vi "S4GUI.vi"() -> ()   [LabVIEW 2018] (continued)
                n1589 = call-dynamic "Write Interface.vi"("error in (no error)"=w3557, "Interface.lvclass"=w3544, "Channel in"=w3552) -> ("error out"=w3525:errorcluster, "Channel out"=w3524:refnum<class "Channel.lvclass">)  [unwired: 7 in]
                n1590 = call-dynamic "Write ciclos.vi"("error in (no error)"=w3525, "ciclos"=w3523, "Channel in"=w3524) -> ("error out"=w3521:errorcluster, "Channel out"=w3522:refnum<class "Channel.lvclass">)  [unwired: 7 in]
                n1591 = call-dynamic "Write sequencias.vi"("error in (no error)"=w3521, "sequencias"=w3518, "Channel in"=w3522) -> ("error out"=w3520:errorcluster, "Channel out"=w3519:refnum<class "Channel.lvclass">)  [unwired: 7 in]
                n1592 = call-dynamic "Write Channel.vi"("error in (no error)"=w3520, "Channel.lvclass"=w3519, "Acquisition in"=w3542) -> ("error out"=w3540:errorcluster, "Acquisition out"=w3541:refnum<class "Acquisition.lvclass">)  [unwired: 7 in]
                n1593 = call-dynamic "Write AcquisitionD.vi"("error in (no error)"=w3540, "Acquisition.lvclass"=w3541, "S4ACS_GUI in"=w3543) -> ("error out"=w3566:errorcluster, "S4ACS_GUI out"=w3567:refnum<class "S4GUI.lvclass">)  [unwired: 7 in]
              }
            }
            n1594 = call-dynamic "Write sequencias.vi"("error in (no error)"=w3342, "sequencias"=w3338, "S4GUI in"=w3340) -> ("error out"=w3341:errorcluster, "S4GUI out"=w3339:refnum<class "S4GUI.lvclass">)  [unwired: 7 in]
            n1595 = call-dynamic "Write ciclos.vi"("error in (no error)"=w3341, "ciclos"=w3343, "S4ACS_GUI in"=w3339) -> ("error out"=w3345:errorcluster, "S4ACS_GUI out"=w3347:refnum<class "S4GUI.lvclass">)  [unwired: 7 in]
            n1596 = property on="#Cycles Done" class="Slide (strict)"("Scale.Maximum"=w3343, "Scale.Minimum"=0.0 ("Scale.Range:Minor Increment")) -> ()  [unwired: 2 in, 2 out]
            n1597 = call-dynamic "Write TotalCiclos.vi"("error in (no error)"=w3345, "TotalCiclos"=w3343, "S4GUI in"=w3347) -> ("error out"=w3344:errorcluster, "S4GUI out"=w3346:refnum<class "S4GUI.lvclass">)  [unwired: 7 in]
          }
        }
        n1598 = property on="Pause SM" class="Bool"(error in=w3207, "DisabledEnum"=T7."Enabled" ("Disabled")) -> (error out=w3206:errorcluster)  [unwired: 1 in, 1 out]
      }
      event "# Cycles": Value Change {
        n1599 = event-data() -> ("NewVal"=w3572:u32)  [unwired: 1 in]
        n1600 = call-dynamic "Write ciclos.vi"("error in (no error)"=w3573, "ciclos"=w3572, "S4ACS_GUI in"=w3574) -> ("error out"=w3571:errorcluster, "S4ACS_GUI out"=w3570:refnum<class "S4GUI.lvclass">)  [unwired: 7 in]
        n1601 = property on="#Cycles Done" class="Slide (strict)"("Scale.Maximum"=w3572, "Scale.Minimum"=0.0 ("Scale.Range:Minor Increment")) -> ()  [unwired: 2 in, 2 out]
      }
      event "AllConfig": Value Change {
        n1602 = event-data() -> ()  [unwired: 1 in, 6 out]
        n1603 = call "Read Instrument.lvclass.vi"("error in (no error)"=w3580, "S4ACS_GUI in"=w3581) -> ("error out"=w3660:errorcluster, "Instrument.lvclass"=w3627:refnum<class "Instrument.lvclass">, "S4ACS_GUI out"=w3658:refnum<class "S4GUI.lvclass">)  [unwired: 7 in]
        n1604 = call "Read ASEL.vi"("error in (no error)"=w3660, "Instrument in"=w3627) -> ("error out"=w3652:errorcluster, "Opt_Selector.lvclass"=w3651:refnum<class "Opt_Selector.lvclass">, "Instrument out"=w3659:refnum<class "Instrument.lvclass">)  [unwired: 7 in]
        n1605 = call-dynamic "Read State Machine.vi"("error in (no error)"=w3652, "Device in"=w3651) -> ("error out"=w3655:errorcluster, "State Machine.lvclass"=w3657:refnum<class "State Machine.lvclass">, "Device out"=w3649:refnum<class "Opt_Selector.lvclass">)  [unwired: 7 in]
        n1606 = call "Next State.vi"("error in (no error)"=w3655, "New_State"=1, "State Machine in"=w3657) -> ("error out"=w3654:errorcluster, "State Machine out"=w3653:refnum<class "State Machine.lvclass">)  [unwired: 7 in]
        n1607 = call-dynamic "Write State Machine.vi"("error in (no error)"=w3654, "State Machine.lvclass"=w3653, "Device in"=w3649) -> ("error out"=w3648:errorcluster, "Device out"=w3650:refnum<class "Opt_Selector.lvclass">)  [unwired: 7 in]
        n1608 = call "Write ASEL.vi"("error in (no error)"=w3648, "Opt_Selector.lvclass"=w3650, "Instrument in"=w3659) -> ("error out"=w3610:errorcluster, "Instrument out"=w3626:refnum<class "Instrument.lvclass">)  [unwired: 7 in]
        n1609 = call "Read CALW.vi"("error in (no error)"=w3610, "Instrument in"=w3626) -> ("error out"=w3643:errorcluster, "Opt_Selector.lvclass"=w3644:refnum<class "Opt_Selector.lvclass">, "Instrument out"=w3625:refnum<class "Instrument.lvclass">)  [unwired: 7 in]
        n1610 = call-dynamic "Read State Machine.vi"("error in (no error)"=w3643, "Device in"=w3644) -> ("error out"=w3640:errorcluster, "State Machine.lvclass"=w3638:refnum<class "State Machine.lvclass">, "Device out"=w3646:refnum<class "Opt_Selector.lvclass">)  [unwired: 7 in]
        n1611 = call "Next State.vi"("error in (no error)"=w3640, "New_State"=1, "State Machine in"=w3638) -> ("error out"=w3641:errorcluster, "State Machine out"=w3642:refnum<class "State Machine.lvclass">)  [unwired: 7 in]
        n1612 = call-dynamic "Write State Machine.vi"("error in (no error)"=w3641, "State Machine.lvclass"=w3642, "Device in"=w3646) -> ("error out"=w3647:errorcluster, "Device out"=w3645:refnum<class "Opt_Selector.lvclass">)  [unwired: 7 in]
        n1613 = call "Write CALW.vi"("error in (no error)"=w3647, "Opt_Selector.lvclass"=w3645, "Instrument in"=w3625) -> ("error out"=w3609:errorcluster, "Instrument out"=w3624:refnum<class "Instrument.lvclass">)  [unwired: 7 in]
        n1614 = call "Read WPSEL.vi"("error in (no error)"=w3609, "Instrument in"=w3624) -> ("error out"=w3632:errorcluster, "Opt_Selector.lvclass"=w3631:refnum<class "Opt_Selector.lvclass">, "Instrument out"=w3623:refnum<class "Instrument.lvclass">)  [unwired: 7 in]
        n1615 = call-dynamic "Read State Machine.vi"("error in (no error)"=w3632, "Device in"=w3631) -> ("error out"=w3635:errorcluster, "State Machine.lvclass"=w3637:refnum<class "State Machine.lvclass">, "Device out"=w3629:refnum<class "Opt_Selector.lvclass">)  [unwired: 7 in]
        n1616 = call "Next State.vi"("error in (no error)"=w3635, "New_State"=1, "State Machine in"=w3637) -> ("error out"=w3634:errorcluster, "State Machine out"=w3633:refnum<class "State Machine.lvclass">)  [unwired: 7 in]
        n1617 = call-dynamic "Write State Machine.vi"("error in (no error)"=w3634, "State Machine.lvclass"=w3633, "Device in"=w3629) -> ("error out"=w3628:errorcluster, "Device out"=w3630:refnum<class "Opt_Selector.lvclass">)  [unwired: 7 in]
        n1618 = call "Write WPSEL.vi"("error in (no error)"=w3628, "Opt_Selector.lvclass"=w3630, "Instrument in"=w3623) -> ("error out"=w3608:errorcluster, "Instrument out"=w3612:refnum<class "Instrument.lvclass">)  [unwired: 7 in]
        n1619 = call "Read WPROT.vi"("error in (no error)"=w3608, "Instrument in"=w3612) -> ("error out"=w3618:errorcluster, "Opt_Selector.lvclass"=w3619:refnum<class "Opt_Selector.lvclass">, "Instrument out"=w3611:refnum<class "Instrument.lvclass">)  [unwired: 7 in]
        n1620 = call-dynamic "Read State Machine.vi"("error in (no error)"=w3618, "Device in"=w3619) -> ("error out"=w3615:errorcluster, "State Machine.lvclass"=w3613:refnum<class "State Machine.lvclass">, "Device out"=w3621:refnum<class "Opt_Selector.lvclass">)  [unwired: 7 in]
        n1621 = call "Next State.vi"("error in (no error)"=w3615, "New_State"=1, "State Machine in"=w3613) -> ("error out"=w3616:errorcluster, "State Machine out"=w3617:refnum<class "State Machine.lvclass">)  [unwired: 7 in]
        n1622 = call-dynamic "Write State Machine.vi"("error in (no error)"=w3616, "State Machine.lvclass"=w3617, "Device in"=w3621) -> ("error out"=w3622:errorcluster, "Device out"=w3620:refnum<class "Opt_Selector.lvclass">)  [unwired: 7 in]
        n1623 = call "Write WPROT.vi"("error in (no error)"=w3622, "Opt_Selector.lvclass"=w3620, "Instrument in"=w3611) -> ("error out"=w3584:errorcluster, "Instrument out"=w3585:refnum<class "Instrument.lvclass">)  [unwired: 7 in]
        n1624 = call "Read GMIR.vi"("error in (no error)"=w3584, "Instrument in"=w3585) -> ("error out"=w3603:errorcluster, "Opt_Continuous.lvclass"=w3604:refnum<class "Opt_Continuous.lvclass">, "Instrument out"=w3597:refnum<class "Instrument.lvclass">)  [unwired: 7 in]
        n1625 = call-dynamic "Read State Machine.vi"("error in (no error)"=w3603, "Device in"=w3604) -> ("error out"=w3600:errorcluster, "State Machine.lvclass"=w3598:refnum<class "State Machine.lvclass">, "Device out"=w3606:refnum<class "Opt_Continuous.lvclass">)  [unwired: 7 in]
        n1626 = call "Next State.vi"("error in (no error)"=w3600, "New_State"=1, "State Machine in"=w3598) -> ("error out"=w3601:errorcluster, "State Machine out"=w3602:refnum<class "State Machine.lvclass">)  [unwired: 7 in]
        n1627 = call-dynamic "Write State Machine.vi"("error in (no error)"=w3601, "State Machine.lvclass"=w3602, "Device in"=w3606) -> ("error out"=w3607:errorcluster, "Device out"=w3605:refnum<class "Opt_Continuous.lvclass">)  [unwired: 7 in]
        n1628 = call "Write GMIR.vi"("error in (no error)"=w3607, "Opt_Continuous.lvclass"=w3605, "Instrument in"=w3597) -> ("error out"=w3582:errorcluster, "Instrument out"=w3583:refnum<class "Instrument.lvclass">)  [unwired: 7 in]
        n1629 = call "Read GFOC.vi"("error in (no error)"=w3582, "Instrument in"=w3583) -> ("error out"=w3592:errorcluster, "Opt_Continuous.lvclass"=w3593:refnum<class "Opt_Continuous.lvclass">, "Instrument out"=w3586:refnum<class "Instrument.lvclass">)  [unwired: 7 in]
        n1630 = call-dynamic "Read State Machine.vi"("error in (no error)"=w3592, "Device in"=w3593) -> ("error out"=w3589:errorcluster, "State Machine.lvclass"=w3587:refnum<class "State Machine.lvclass">, "Device out"=w3595:refnum<class "Opt_Continuous.lvclass">)  [unwired: 7 in]
        n1631 = call "Next State.vi"("error in (no error)"=w3589, "New_State"=1, "State Machine in"=w3587) -> ("error out"=w3590:errorcluster, "State Machine out"=w3591:refnum<class "State Machine.lvclass">)  [unwired: 7 in]
        n1632 = call-dynamic "Write State Machine.vi"("error in (no error)"=w3590, "State Machine.lvclass"=w3591, "Device in"=w3595) -> ("error out"=w3596:errorcluster, "Device out"=w3594:refnum<class "Opt_Continuous.lvclass">)  [unwired: 7 in]
        n1633 = call "Write GFOC.vi"("error in (no error)"=w3596, "Opt_Continuous.lvclass"=w3594, "Instrument in"=w3586) -> ("error out"=w3578:errorcluster, "Instrument out"=w3579:refnum<class "Instrument.lvclass">)  [unwired: 7 in]
        n1634 = call "Write Instrument.lvclass.vi"("error in (no error)"=w3578, "Instrument.lvclass"=w3579, "S4ACS_GUI in"=w3658) -> ("error out"=w3577:errorcluster, "S4ACS_GUI out"=w3576:refnum<class "S4GUI.lvclass">)  [unwired: 7 in]
      }
      event "Tab Acq Type": Value Change {
        # "Tab for choosing EXPOSURE MODE: Object, Dflat, Sflat, Dark, Zero, Focus"
        n1635 = event-data() -> ("NewVal"=w3667:T1)  [unwired: 1 in]
        n1636 = local read "Observer"() -> (w3662:string)
        n1637 = case shown="\"OBJECT\", Default" w3667 {
          tunnel: ["OBJECT" "FLAT" "FLAT" "DARK" "ZERO" "FOCUS"] -> w3666
          tunnel: [w3703 w3707 w3711 w3715 w3719 w3723] -> w3665
          tunnel: [w3702 w3706 w3710 w3714 w3718 w3722] -> w3664
          tunnel: [w3701 w3705 w3709 w3713 w3717 w3721] -> w3663
          frame "OBJECT", Default {
            n1638 = local read "Object_obj"() -> (w3703:string)
            n1639 = local read "OBJECT Comments"() -> (w3701:string)
            n1640 = local read "object suffix"() -> (w3702:string)
          }
          frame "DFLAT" {
            n1641 = local read "DFLAT Comments"() -> (w3705:string)
            n1642 = local read "Object_dflat"() -> (w3707:string)
            n1643 = local read "dflat suffix"() -> (w3706:string)
          }
          frame "SFLAT" {
            n1644 = local read "SFLAT Comments"() -> (w3709:string)
            n1645 = local read "Object_sflat"() -> (w3711:string)
            n1646 = local read "sflat suffix"() -> (w3710:string)
          }
          frame "DARK" {
            n1647 = local read "Object_dark"() -> (w3715:string)
            n1648 = local read "dark suffix"() -> (w3714:string)
            n1649 = local read "DARK Comments"() -> (w3713:string)
          }
          frame "ZERO" {
            n1650 = local read "ZERO Comments"() -> (w3717:string)
            n1651 = local read "Object_zero"() -> (w3719:string)
            n1652 = local read "zero suffix"() -> (w3718:string)
          }
          frame "FOCUS" {
            n1653 = local read "FOCUS Comments"() -> (w3721:string)
            n1654 = local read "Object_focus"() -> (w3723:string)
            n1655 = local read "focus suffix"() -> (w3722:string)
          }
        }
        n1656 = call-dynamic "Write ExpMode.vi"("error in (no error)"=w3670, "ExpMode"=w3667, "S4GUI in"=w3671) -> ("error out"=w3668:errorcluster, "S4GUI out"=w3669:refnum<class "S4GUI.lvclass">)  [unwired: 7 in]
        n1657 = call-dynamic "Read AcquisitionC.vi"("error in (no error)"=w3668, "S4ACS_GUI in"=w3669) -> ("error out"=w3674:errorcluster, "Acquisition.lvclass"=w3675:refnum<class "Acquisition.lvclass">)  [unwired: 7 in, 1 out]
        n1658 = call-dynamic "Read AcquisitionA.vi"("error in (no error)"=w3668, "S4ACS_GUI in"=w3669) -> ("error out"=w3678:errorcluster, "Acquisition.lvclass"=w3679:refnum<class "Acquisition.lvclass">, "S4ACS_GUI out"=w3700:refnum<class "S4GUI.lvclass">)  [unwired: 7 in]
        n1659 = call "Read AcquisitionB.vi"("error in (no error)"=w3668, "S4ACS_GUI in"=w3669) -> ("error out"=w3676:errorcluster, "Acquisition.lvclass"=w3677:refnum<class "Acquisition.lvclass">)  [unwired: 7 in, 1 out]
        n1660 = call-dynamic "Read AcquisitionD.vi"("error in (no error)"=w3668, "S4ACS_GUI in"=w3669) -> ("error out"=w3672:errorcluster, "Acquisition.lvclass"=w3673:refnum<class "Acquisition.lvclass">)  [unwired: 7 in, 1 out]
        n1661 = To Lower Case(string=w3664) -> (all lower case string=w3661:string)
        n1662 = case shown="\"OBJECT\", Default" w3667 {
          tunnel: [w3753 w3942 w4136] -> w3699
          tunnel: [w3752 w3941 w4135] -> w3698
          tunnel: [w3751 w3940 w4134] -> w3694
          tunnel: [w3750 w3939 w4133] -> w3693
          tunnel: [w3749 w3938 w4132] -> w3683
          tunnel: [w3748 w3937 w4131] -> w3682
          tunnel: [w3747 w3936 w4130] -> w3681
          tunnel: [w3746 w3935 w4129] -> w3680
          tunnel: w3679 -> [w3745 w3934 w4128]
          tunnel: w3678 -> [w3744 w3933 w4127]
          tunnel: w3677 -> [w3730 w3920 w4114]
          tunnel: w3676 -> [w3729 w3919 w4113]
          tunnel: w3675 -> [w3728 w3918 w4112]
          tunnel: w3674 -> [w3727 w3917 w4111]
          tunnel: w3673 -> [w3726 w3916 w4110]
          tunnel: w3672 -> [w3725 w3915 w4109]
          tunnel: w3661 -> [_ _ w4108]
          tunnel: w3666 -> [_ _ w4107]
          tunnel: w3665 -> [_ _ w4106]
          tunnel: w3663 -> [_ _ w4105]
          tunnel: w3662 -> [_ _ w4104]
          frame "ZERO" {
            w3743 = 1e-05 ("Exptime ch1")
            # "ZERO: EXPTIME=1E-5 (mandatory) and shutter automatically closed."
            n1663 = call "Read connection.vi"("error in (no error)"=w3725, "Server in"=w3726) -> ("error out"=w3732:errorcluster, "connection"=w3731:bool, "Server out"=w3733:refnum<class "Acquisition.lvclass">)  [unwired: 7 in]
            n1664 = call "Read connection.vi"("error in (no error)"=w3727, "Server in"=w3728) -> ("error out"=w3735:errorcluster, "connection"=w3734:bool, "Server out"=w3736:refnum<class "Acquisition.lvclass">)  [unwired: 7 in]
            n1665 = call "Read connection.vi"("error in (no error)"=w3729, "Server in"=w3730) -> ("error out"=w3738:errorcluster, "connection"=w3737:bool, "Server out"=w3739:refnum<class "Acquisition.lvclass">)  [unwired: 7 in]
            n1666 = call "Read connection.vi"("error in (no error)"=w3744, "Server in"=w3745) -> ("error out"=w3741:errorcluster, "connection"=w3740:bool, "Server out"=w3742:refnum<class "Acquisition.lvclass">)  [unwired: 7 in]
            n1667 = case shown="True" w3737 {
              tunnel: w3739 -> [w3838 w3842]
              tunnel: w3738 -> [w3837 w3841]
              tunnel: [w3838 w3840] -> w3751
              tunnel: [w3837 w3839] -> w3750
              frame False {
              }
              frame True {
                # "nome do arquivo .cfg"
                # "seção no arquivo .cfg"
                # "closed"
                n1668 = call-dynamic "Read Channel.vi"("error in (no error)"=w3841, "Acquisition in"=w3842) -> ("error out"=w3846:errorcluster, "Channel.lvclass"=w3845:refnum<class "Channel.lvclass">, "Acquisition out"=w3844:refnum<class "Acquisition.lvclass">)  [unwired: 7 in]
                n1669 = call-dynamic "Read Interface.vi"("error in (no error)"=w3846, "Channel in"=w3845) -> ("error out"=w3854:errorcluster, "Interface.lvclass"=w3855:refnum<class "Interface.lvclass">, "Channel out"=w3843:refnum<class "Channel.lvclass">)  [unwired: 7 in]
                n1670 = call-dynamic "Get CCD_Config.vi"("error in (no error)"=w3854, "Interface in"=w3855) -> ("error out"=w3851:errorcluster, "output cluster"=w3850:T24, "Interface out"=w3856:refnum<class "Interface.lvclass">)  [unwired: 7 in]
                n1671 = Bundle By Name(cluster=w3850, "SHUTTER_MODE"=u8 2) -> (w3852:T24)
                n1672 = call-dynamic "Set CCD_Config.vi"("error in (no error)"=w3851, "input cluster"=w3852, "Interface in"=w3856) -> ("error out"=w3849:errorcluster, "Interface out"=w3857:refnum<class "Interface.lvclass">)  [unwired: 7 in]
                n1673 = Flatten To String(anything=w3852, error in (no error)=w3849) -> (data string=w3847:string, error out=w3848:errorcluster)  [unwired: 2 in, 1 out]
                n1674 = call "Write flatted cluster.vi"("error in (no error)"=w3848, "flatted cluster"=w3847, "Interface in"=w3857) -> ("error out"=w3859:errorcluster, "Interface out"=w3858:refnum<class "Interface.lvclass">)  [unwired: 7 in]
                n1675 = call-dynamic "Write Interface.vi"("error in (no error)"=w3859, "Interface.lvclass"=w3858, "Channel in"=w3843) -> ("error out"=w3865:errorcluster, "Channel out"=w3866:refnum<class "Channel.lvclass">)  [unwired: 7 in]
                n1676 = call "Write section_name.vi"("error in (no error)"=w3865, "section_name"="CCD_ACS2", "Channel in"=w3866) -> ("error out"=w3863:errorcluster, "Channel out"=w3869:refnum<class "Channel.lvclass">)  [unwired: 7 in]
                n1677 = call-dynamic "save config.vi"("error in (no error)"=w3863, "file config"="lastsaved.cfg", "Channel in"=w3869) -> ("error out"=w3864:errorcluster, "Channel out"=w3870:refnum<class "Channel.lvclass">)  [unwired: 7 in]
                n1678 = call-dynamic "Read State Machine.vi"("error in (no error)"=w3864, "Device in"=w3870) -> ("error out"=w3860:errorcluster, "State Machine.lvclass"=w3872:refnum<class "State Machine.lvclass">, "Device out"=w3871:refnum<class "Channel.lvclass">)  [unwired: 7 in]
                n1679 = call-dynamic "Write State.vi"("error in (no error)"=w3860, "State"=60, "State Machine in"=w3872) -> ("error out"=w3861:errorcluster, "State Machine out"=w3873:refnum<class "State Machine.lvclass">)  [unwired: 7 in]
                n1680 = call-dynamic "Write State Machine.vi"("error in (no error)"=w3861, "State Machine.lvclass"=w3873, "Device in"=w3871) -> ("error out"=w3875:errorcluster, "Device out"=w3874:refnum<class "Channel.lvclass">)  [unwired: 7 in]
                n1681 = call-dynamic "Write Channel.vi"("error in (no error)"=w3875, "Channel.lvclass"=w3874, "Acquisition in"=w3844) -> ("error out"=w3839:errorcluster, "Acquisition out"=w3840:refnum<class "Acquisition.lvclass">)  [unwired: 7 in]
              }
            }
            n1682 = case shown="True" w3740 {
              tunnel: [w3876 w3910] -> w3752
              tunnel: [w3877 w3909] -> w3753
              tunnel: w3742 -> [w3877 w3879]
              tunnel: w3741 -> [w3876 w3878]
              frame False {
              }
              frame True {
                # "nome do arquivo .cfg"
                # "seção no arquivo .cfg"
                # "closed"
                n1683 = call-dynamic "Read Channel.vi"("error in (no error)"=w3878, "Acquisition in"=w3879) -> ("error out"=w3911:errorcluster, "Channel.lvclass"=w3912:refnum<class "Channel.lvclass">, "Acquisition out"=w3913:refnum<class "Acquisition.lvclass">)  [unwired: 7 in]
                n1684 = call-dynamic "Read Interface.vi"("error in (no error)"=w3911, "Channel in"=w3912) -> ("error out"=w3901:errorcluster, "Interface.lvclass"=w3900:refnum<class "Interface.lvclass">, "Channel out"=w3914:refnum<class "Channel.lvclass">)  [unwired: 7 in]
                n1685 = call-dynamic "Get CCD_Config.vi"("error in (no error)"=w3901, "Interface in"=w3900) -> ("error out"=w3904:errorcluster, "output cluster"=w3905:T24, "Interface out"=w3899:refnum<class "Interface.lvclass">)  [unwired: 7 in]
                n1686 = Bundle By Name(cluster=w3905, "SHUTTER_MODE"=u8 2) -> (w3903:T24)
                n1687 = call-dynamic "Set CCD_Config.vi"("error in (no error)"=w3904, "input cluster"=w3903, "Interface in"=w3899) -> ("error out"=w3906:errorcluster, "Interface out"=w3898:refnum<class "Interface.lvclass">)  [unwired: 7 in]
                n1688 = Flatten To String(anything=w3903, error in (no error)=w3906) -> (data string=w3908:string, error out=w3907:errorcluster)  [unwired: 2 in, 1 out]
                n1689 = call "Write flatted cluster.vi"("error in (no error)"=w3907, "flatted cluster"=w3908, "Interface in"=w3898) -> ("error out"=w3896:errorcluster, "Interface out"=w3897:refnum<class "Interface.lvclass">)  [unwired: 7 in]
                n1690 = call-dynamic "Write Interface.vi"("error in (no error)"=w3896, "Interface.lvclass"=w3897, "Channel in"=w3914) -> ("error out"=w3891:errorcluster, "Channel out"=w3890:refnum<class "Channel.lvclass">)  [unwired: 7 in]
                n1691 = call "Write section_name.vi"("error in (no error)"=w3891, "section_name"="CCD_ACS1", "Channel in"=w3890) -> ("error out"=w3892:errorcluster, "Channel out"=w3887:refnum<class "Channel.lvclass">)  [unwired: 7 in]
                n1692 = call-dynamic "save config.vi"("error in (no error)"=w3892, "file config"="lastsaved.cfg", "Channel in"=w3887) -> ("error out"=w3880:errorcluster, "Channel out"=w3881:refnum<class "Channel.lvclass">)  [unwired: 7 in]
                n1693 = call-dynamic "Read State Machine.vi"("error in (no error)"=w3880, "Device in"=w3881) -> ("error out"=w3895:errorcluster, "State Machine.lvclass"=w3885:refnum<class "State Machine.lvclass">, "Device out"=w3886:refnum<class "Channel.lvclass">)  [unwired: 7 in]
                n1694 = call-dynamic "Write State.vi"("error in (no error)"=w3895, "State"=60, "State Machine in"=w3885) -> ("error out"=w3894:errorcluster, "State Machine out"=w3884:refnum<class "State Machine.lvclass">)  [unwired: 7 in]
                n1695 = call-dynamic "Write State Machine.vi"("error in (no error)"=w3894, "State Machine.lvclass"=w3884, "Device in"=w3886) -> ("error out"=w3882:errorcluster, "Device out"=w3883:refnum<class "Channel.lvclass">)  [unwired: 7 in]
                n1696 = call-dynamic "Write Channel.vi"("error in (no error)"=w3882, "Channel.lvclass"=w3883, "Acquisition in"=w3913) -> ("error out"=w3910:errorcluster, "Acquisition out"=w3909:refnum<class "Acquisition.lvclass">)  [unwired: 7 in]
              }
            }
            n1697 = case shown="True" w3734 {
              tunnel: w3736 -> [w3799 w3803]
              tunnel: w3735 -> [w3798 w3802]
              tunnel: [w3799 w3801] -> w3749
              tunnel: [w3798 w3800] -> w3748
              frame False {
              }
              frame True {
                # "nome do arquivo .cfg"
                # "seção no arquivo .cfg"
                # "closed"
                n1698 = call-dynamic "Read Channel.vi"("error in (no error)"=w3802, "Acquisition in"=w3803) -> ("error out"=w3807:errorcluster, "Channel.lvclass"=w3806:refnum<class "Channel.lvclass">, "Acquisition out"=w3805:refnum<class "Acquisition.lvclass">)  [unwired: 7 in]
                n1699 = call-dynamic "Read Interface.vi"("error in (no error)"=w3807, "Channel in"=w3806) -> ("error out"=w3815:errorcluster, "Interface.lvclass"=w3816:refnum<class "Interface.lvclass">, "Channel out"=w3804:refnum<class "Channel.lvclass">)  [unwired: 7 in]
                n1700 = call-dynamic "Get CCD_Config.vi"("error in (no error)"=w3815, "Interface in"=w3816) -> ("error out"=w3812:errorcluster, "output cluster"=w3811:T24, "Interface out"=w3817:refnum<class "Interface.lvclass">)  [unwired: 7 in]
                n1701 = Bundle By Name(cluster=w3811, "SHUTTER_MODE"=u8 2) -> (w3813:T24)
                n1702 = call-dynamic "Set CCD_Config.vi"("error in (no error)"=w3812, "input cluster"=w3813, "Interface in"=w3817) -> ("error out"=w3810:errorcluster, "Interface out"=w3818:refnum<class "Interface.lvclass">)  [unwired: 7 in]
                n1703 = Flatten To String(anything=w3813, error in (no error)=w3810) -> (data string=w3808:string, error out=w3809:errorcluster)  [unwired: 2 in, 1 out]
                n1704 = call "Write flatted cluster.vi"("error in (no error)"=w3809, "flatted cluster"=w3808, "Interface in"=w3818) -> ("error out"=w3820:errorcluster, "Interface out"=w3819:refnum<class "Interface.lvclass">)  [unwired: 7 in]
                n1705 = call-dynamic "Write Interface.vi"("error in (no error)"=w3820, "Interface.lvclass"=w3819, "Channel in"=w3804) -> ("error out"=w3826:errorcluster, "Channel out"=w3827:refnum<class "Channel.lvclass">)  [unwired: 7 in]
                n1706 = call "Write section_name.vi"("error in (no error)"=w3826, "section_name"="CCD_ACS3", "Channel in"=w3827) -> ("error out"=w3824:errorcluster, "Channel out"=w3830:refnum<class "Channel.lvclass">)  [unwired: 7 in]
                n1707 = call-dynamic "save config.vi"("error in (no error)"=w3824, "file config"="lastsaved.cfg", "Channel in"=w3830) -> ("error out"=w3825:errorcluster, "Channel out"=w3831:refnum<class "Channel.lvclass">)  [unwired: 7 in]
                n1708 = call-dynamic "Read State Machine.vi"("error in (no error)"=w3825, "Device in"=w3831) -> ("error out"=w3821:errorcluster, "State Machine.lvclass"=w3833:refnum<class "State Machine.lvclass">, "Device out"=w3832:refnum<class "Channel.lvclass">)  [unwired: 7 in]
                n1709 = call-dynamic "Write State.vi"("error in (no error)"=w3821, "State"=60, "State Machine in"=w3833) -> ("error out"=w3822:errorcluster, "State Machine out"=w3834:refnum<class "State Machine.lvclass">)  [unwired: 7 in]
                n1710 = call-dynamic "Write State Machine.vi"("error in (no error)"=w3822, "State Machine.lvclass"=w3834, "Device in"=w3832) -> ("error out"=w3836:errorcluster, "Device out"=w3835:refnum<class "Channel.lvclass">)  [unwired: 7 in]
                n1711 = call-dynamic "Write Channel.vi"("error in (no error)"=w3836, "Channel.lvclass"=w3835, "Acquisition in"=w3805) -> ("error out"=w3800:errorcluster, "Acquisition out"=w3801:refnum<class "Acquisition.lvclass">)  [unwired: 7 in]
              }
            }
            n1712 = case shown="True" w3731 {
              tunnel: w3733 -> [w3760 w3764]
              tunnel: w3732 -> [w3759 w3763]
              tunnel: [w3760 w3762] -> w3747
              tunnel: [w3759 w3761] -> w3746
              frame False {
              }
              frame True {
                # "nome do arquivo .cfg"
                # "seção no arquivo .cfg"
                # "closed"
                n1713 = call-dynamic "Read Channel.vi"("error in (no error)"=w3763, "Acquisition in"=w3764) -> ("error out"=w3794:errorcluster, "Channel.lvclass"=w3795:refnum<class "Channel.lvclass">, "Acquisition out"=w3796:refnum<class "Acquisition.lvclass">)  [unwired: 7 in]
                n1714 = call-dynamic "Read Interface.vi"("error in (no error)"=w3794, "Channel in"=w3795) -> ("error out"=w3786:errorcluster, "Interface.lvclass"=w3785:refnum<class "Interface.lvclass">, "Channel out"=w3797:refnum<class "Channel.lvclass">)  [unwired: 7 in]
                n1715 = call-dynamic "Get CCD_Config.vi"("error in (no error)"=w3786, "Interface in"=w3785) -> ("error out"=w3789:errorcluster, "output cluster"=w3790:T24, "Interface out"=w3784:refnum<class "Interface.lvclass">)  [unwired: 7 in]
                n1716 = Bundle By Name(cluster=w3790, "SHUTTER_MODE"=u8 2) -> (w3788:T24)
                n1717 = call-dynamic "Set CCD_Config.vi"("error in (no error)"=w3789, "input cluster"=w3788, "Interface in"=w3784) -> ("error out"=w3791:errorcluster, "Interface out"=w3783:refnum<class "Interface.lvclass">)  [unwired: 7 in]
                n1718 = Flatten To String(anything=w3788, error in (no error)=w3791) -> (data string=w3793:string, error out=w3792:errorcluster)  [unwired: 2 in, 1 out]
                n1719 = call "Write flatted cluster.vi"("error in (no error)"=w3792, "flatted cluster"=w3793, "Interface in"=w3783) -> ("error out"=w3781:errorcluster, "Interface out"=w3782:refnum<class "Interface.lvclass">)  [unwired: 7 in]
                n1720 = call-dynamic "Write Interface.vi"("error in (no error)"=w3781, "Interface.lvclass"=w3782, "Channel in"=w3797) -> ("error out"=w3775:errorcluster, "Channel out"=w3774:refnum<class "Channel.lvclass">)  [unwired: 7 in]
                n1721 = call "Write section_name.vi"("error in (no error)"=w3775, "section_name"="CCD_ACS4", "Channel in"=w3774) -> ("error out"=w3777:errorcluster, "Channel out"=w3771:refnum<class "Channel.lvclass">)  [unwired: 7 in]
                n1722 = call-dynamic "save config.vi"("error in (no error)"=w3777, "file config"="lastsaved.cfg", "Channel in"=w3771) -> ("error out"=w3776:errorcluster, "Channel out"=w3770:refnum<class "Channel.lvclass">)  [unwired: 7 in]
                n1723 = call-dynamic "Read State Machine.vi"("error in (no error)"=w3776, "Device in"=w3770) -> ("error out"=w3780:errorcluster, "State Machine.lvclass"=w3768:refnum<class "State Machine.lvclass">, "Device out"=w3769:refnum<class "Channel.lvclass">)  [unwired: 7 in]
                n1724 = call-dynamic "Write State.vi"("error in (no error)"=w3780, "State"=60, "State Machine in"=w3768) -> ("error out"=w3779:errorcluster, "State Machine out"=w3767:refnum<class "State Machine.lvclass">)  [unwired: 7 in]
                n1725 = call-dynamic "Write State Machine.vi"("error in (no error)"=w3779, "State Machine.lvclass"=w3767, "Device in"=w3769) -> ("error out"=w3765:errorcluster, "Device out"=w3766:refnum<class "Channel.lvclass">)  [unwired: 7 in]
                n1726 = call-dynamic "Write Channel.vi"("error in (no error)"=w3765, "Channel.lvclass"=w3766, "Acquisition in"=w3796) -> ("error out"=w3761:errorcluster, "Acquisition out"=w3762:refnum<class "Acquisition.lvclass">)  [unwired: 7 in]
              }
            }
            n1727 = property on="Exptime ch1" class="DigNum (strict)"("Value"=w3743) -> ()  [unwired: 2 in, 2 out]
            n1728 = property on="Exptime ch2" class="DigNum (strict)"("Value"=w3743) -> ()  [unwired: 2 in, 2 out]
            n1729 = property on="Exptime ch3" class="DigNum (strict)"("Value"=w3743) -> ()  [unwired: 2 in, 2 out]
            n1730 = property on="Exptime ch4" class="DigNum (strict)"("Value"=w3743) -> ()  [unwired: 2 in, 2 out]
            n1731 = disable-structure shown="Enabled" {
              frame Disabled {
                # "closed"
                n1732 = local read "Input Cluster"() -> (w3756:T5)
                n1733 = Unbundle By Name(w3756) -> ("Parameters"=w3757:T23)
                n1734 = Bundle By Name(cluster=w3757, "Shutter\nMode"=u16 2 ("Shutter\nMode")) -> (w3754:T23)
                n1735 = Bundle By Name(cluster=w3756, "Parameters"=w3754) -> (w3755:T5)
                n1736 = local write "Input Cluster"(w3755) -> ()
              }
              frame Enabled {
              }
            }
          }
          frame "DARK" {
            # "DARK: Shutter automatically closed."
            n1737 = call "Read connection.vi"("error in (no error)"=w3915, "Server in"=w3916) -> ("error out"=w3922:errorcluster, "connection"=w3921:bool, "Server out"=w3923:refnum<class "Acquisition.lvclass">)  [unwired: 7 in]
            n1738 = call "Read connection.vi"("error in (no error)"=w3917, "Server in"=w3918) -> ("error out"=w3925:errorcluster, "connection"=w3924:bool, "Server out"=w3926:refnum<class "Acquisition.lvclass">)  [unwired: 7 in]
            n1739 = call "Read connection.vi"("error in (no error)"=w3919, "Server in"=w3920) -> ("error out"=w3928:errorcluster, "connection"=w3927:bool, "Server out"=w3929:refnum<class "Acquisition.lvclass">)  [unwired: 7 in]
            n1740 = call "Read connection.vi"("error in (no error)"=w3933, "Server in"=w3934) -> ("error out"=w3931:errorcluster, "connection"=w3930:bool, "Server out"=w3932:refnum<class "Acquisition.lvclass">)  [unwired: 7 in]
            n1741 = case shown="True" w3927 {
              tunnel: w3929 -> [w4027 w4031]
              tunnel: w3928 -> [w4026 w4030]
              tunnel: [w4027 w4029] -> w3940
              tunnel: [w4026 w4028] -> w3939
              frame False {
              }
              frame True {
                # "nome do arquivo .cfg"
                # "seção no arquivo .cfg"
                # "closed"
                n1742 = call-dynamic "Read Channel.vi"("error in (no error)"=w4030, "Acquisition in"=w4031) -> ("error out"=w4035:errorcluster, "Channel.lvclass"=w4034:refnum<class "Channel.lvclass">, "Acquisition out"=w4033:refnum<class "Acquisition.lvclass">)  [unwired: 7 in]
                n1743 = call-dynamic "Read Interface.vi"("error in (no error)"=w4035, "Channel in"=w4034) -> ("error out"=w4043:errorcluster, "Interface.lvclass"=w4044:refnum<class "Interface.lvclass">, "Channel out"=w4032:refnum<class "Channel.lvclass">)  [unwired: 7 in]
                n1744 = call-dynamic "Get CCD_Config.vi"("error in (no error)"=w4043, "Interface in"=w4044) -> ("error out"=w4040:errorcluster, "output cluster"=w4039:T24, "Interface out"=w4045:refnum<class "Interface.lvclass">)  [unwired: 7 in]
                n1745 = Bundle By Name(cluster=w4039, "SHUTTER_MODE"=u8 2) -> (w4041:T24)
                n1746 = call-dynamic "Set CCD_Config.vi"("error in (no error)"=w4040, "input cluster"=w4041, "Interface in"=w4045) -> ("error out"=w4038:errorcluster, "Interface out"=w4046:refnum<class "Interface.lvclass">)  [unwired: 7 in]
                n1747 = Flatten To String(anything=w4041, error in (no error)=w4038) -> (data string=w4036:string, error out=w4037:errorcluster)  [unwired: 2 in, 1 out]
                n1748 = call "Write flatted cluster.vi"("error in (no error)"=w4037, "flatted cluster"=w4036, "Interface in"=w4046) -> ("error out"=w4048:errorcluster, "Interface out"=w4047:refnum<class "Interface.lvclass">)  [unwired: 7 in]
                n1749 = call-dynamic "Write Interface.vi"("error in (no error)"=w4048, "Interface.lvclass"=w4047, "Channel in"=w4032) -> ("error out"=w4054:errorcluster, "Channel out"=w4055:refnum<class "Channel.lvclass">)  [unwired: 7 in]
                n1750 = call "Write section_name.vi"("error in (no error)"=w4054, "section_name"="CCD_ACS2", "Channel in"=w4055) -> ("error out"=w4052:errorcluster, "Channel out"=w4058:refnum<class "Channel.lvclass">)  [unwired: 7 in]
                n1751 = call-dynamic "save config.vi"("error in (no error)"=w4052, "file config"="lastsaved.cfg", "Channel in"=w4058) -> ("error out"=w4053:errorcluster, "Channel out"=w4059:refnum<class "Channel.lvclass">)  [unwired: 7 in]
                n1752 = call-dynamic "Read State Machine.vi"("error in (no error)"=w4053, "Device in"=w4059) -> ("error out"=w4049:errorcluster, "State Machine.lvclass"=w4061:refnum<class "State Machine.lvclass">, "Device out"=w4060:refnum<class "Channel.lvclass">)  [unwired: 7 in]
                n1753 = call-dynamic "Write State.vi"("error in (no error)"=w4049, "State"=60, "State Machine in"=w4061) -> ("error out"=w4050:errorcluster, "State Machine out"=w4062:refnum<class "State Machine.lvclass">)  [unwired: 7 in]
                n1754 = call-dynamic "Write State Machine.vi"("error in (no error)"=w4050, "State Machine.lvclass"=w4062, "Device in"=w4060) -> ("error out"=w4064:errorcluster, "Device out"=w4063:refnum<class "Channel.lvclass">)  [unwired: 7 in]
                n1755 = call-dynamic "Write Channel.vi"("error in (no error)"=w4064, "Channel.lvclass"=w4063, "Acquisition in"=w4033) -> ("error out"=w4028:errorcluster, "Acquisition out"=w4029:refnum<class "Acquisition.lvclass">)  [unwired: 7 in]
              }
            }
            n1756 = case shown="True" w3930 {
              tunnel: [w4065 w4099] -> w3941
              tunnel: [w4066 w4098] -> w3942
              tunnel: w3932 -> [w4066 w4068]
              tunnel: w3931 -> [w4065 w4067]
              frame False {
              }
              frame True {
                # "nome do arquivo .cfg"
                # "seção no arquivo .cfg"
                # "closed"
                n1757 = call-dynamic "Read Channel.vi"("error in (no error)"=w4067, "Acquisition in"=w4068) -> ("error out"=w4100:errorcluster, "Channel.lvclass"=w4101:refnum<class "Channel.lvclass">, "Acquisition out"=w4102:refnum<class "Acquisition.lvclass">)  [unwired: 7 in]
                n1758 = call-dynamic "Read Interface.vi"("error in (no error)"=w4100, "Channel in"=w4101) -> ("error out"=w4090:errorcluster, "Interface.lvclass"=w4089:refnum<class "Interface.lvclass">, "Channel out"=w4103:refnum<class "Channel.lvclass">)  [unwired: 7 in]
                n1759 = call-dynamic "Get CCD_Config.vi"("error in (no error)"=w4090, "Interface in"=w4089) -> ("error out"=w4093:errorcluster, "output cluster"=w4094:T24, "Interface out"=w4088:refnum<class "Interface.lvclass">)  [unwired: 7 in]
                n1760 = Bundle By Name(cluster=w4094, "SHUTTER_MODE"=u8 2) -> (w4092:T24)
                n1761 = call-dynamic "Set CCD_Config.vi"("error in (no error)"=w4093, "input cluster"=w4092, "Interface in"=w4088) -> ("error out"=w4095:errorcluster, "Interface out"=w4087:refnum<class "Interface.lvclass">)  [unwired: 7 in]
                n1762 = Flatten To String(anything=w4092, error in (no error)=w4095) -> (data string=w4097:string, error out=w4096:errorcluster)  [unwired: 2 in, 1 out]
                n1763 = call "Write flatted cluster.vi"("error in (no error)"=w4096, "flatted cluster"=w4097, "Interface in"=w4087) -> ("error out"=w4085:errorcluster, "Interface out"=w4086:refnum<class "Interface.lvclass">)  [unwired: 7 in]
                n1764 = call-dynamic "Write Interface.vi"("error in (no error)"=w4085, "Interface.lvclass"=w4086, "Channel in"=w4103) -> ("error out"=w4080:errorcluster, "Channel out"=w4079:refnum<class "Channel.lvclass">)  [unwired: 7 in]
                n1765 = call "Write section_name.vi"("error in (no error)"=w4080, "section_name"="CCD_ACS1", "Channel in"=w4079) -> ("error out"=w4081:errorcluster, "Channel out"=w4076:refnum<class "Channel.lvclass">)  [unwired: 7 in]
                n1766 = call-dynamic "save config.vi"("error in (no error)"=w4081, "file config"="lastsaved.cfg", "Channel in"=w4076) -> ("error out"=w4069:errorcluster, "Channel out"=w4070:refnum<class "Channel.lvclass">)  [unwired: 7 in]
                n1767 = call-dynamic "Read State Machine.vi"("error in (no error)"=w4069, "Device in"=w4070) -> ("error out"=w4084:errorcluster, "State Machine.lvclass"=w4074:refnum<class "State Machine.lvclass">, "Device out"=w4075:refnum<class "Channel.lvclass">)  [unwired: 7 in]
                n1768 = call-dynamic "Write State.vi"("error in (no error)"=w4084, "State"=60, "State Machine in"=w4074) -> ("error out"=w4083:errorcluster, "State Machine out"=w4073:refnum<class "State Machine.lvclass">)  [unwired: 7 in]
                n1769 = call-dynamic "Write State Machine.vi"("error in (no error)"=w4083, "State Machine.lvclass"=w4073, "Device in"=w4075) -> ("error out"=w4071:errorcluster, "Device out"=w4072:refnum<class "Channel.lvclass">)  [unwired: 7 in]
                n1770 = call-dynamic "Write Channel.vi"("error in (no error)"=w4071, "Channel.lvclass"=w4072, "Acquisition in"=w4102) -> ("error out"=w4099:errorcluster, "Acquisition out"=w4098:refnum<class "Acquisition.lvclass">)  [unwired: 7 in]
              }
            }
            n1771 = case shown="True" w3924 {
              tunnel: w3926 -> [w3988 w3992]
              tunnel: w3925 -> [w3987 w3991]
              tunnel: [w3988 w3990] -> w3938
              tunnel: [w3987 w3989] -> w3937
              frame False {
              }
              frame True {
                # "nome do arquivo .cfg"
                # "seção no arquivo .cfg"
                # "closed"
                n1772 = call-dynamic "Read Channel.vi"("error in (no error)"=w3991, "Acquisition in"=w3992) -> ("error out"=w3996:errorcluster, "Channel.lvclass"=w3995:refnum<class "Channel.lvclass">, "Acquisition out"=w3994:refnum<class "Acquisition.lvclass">)  [unwired: 7 in]
                n1773 = call-dynamic "Read Interface.vi"("error in (no error)"=w3996, "Channel in"=w3995) -> ("error out"=w4004:errorcluster, "Interface.lvclass"=w4005:refnum<class "Interface.lvclass">, "Channel out"=w3993:refnum<class "Channel.lvclass">)  [unwired: 7 in]
                n1774 = call-dynamic "Get CCD_Config.vi"("error in (no error)"=w4004, "Interface in"=w4005) -> ("error out"=w4001:errorcluster, "output cluster"=w4000:T24, "Interface out"=w4006:refnum<class "Interface.lvclass">)  [unwired: 7 in]
                n1775 = Bundle By Name(cluster=w4000, "SHUTTER_MODE"=u8 2) -> (w4002:T24)
                n1776 = call-dynamic "Set CCD_Config.vi"("error in (no error)"=w4001, "input cluster"=w4002, "Interface in"=w4006) -> ("error out"=w3999:errorcluster, "Interface out"=w4007:refnum<class "Interface.lvclass">)  [unwired: 7 in]
                n1777 = Flatten To String(anything=w4002, error in (no error)=w3999) -> (data string=w3997:string, error out=w3998:errorcluster)  [unwired: 2 in, 1 out]
                n1778 = call "Write flatted cluster.vi"("error in (no error)"=w3998, "flatted cluster"=w3997, "Interface in"=w4007) -> ("error out"=w4009:errorcluster, "Interface out"=w4008:refnum<class "Interface.lvclass">)  [unwired: 7 in]
                n1779 = call-dynamic "Write Interface.vi"("error in (no error)"=w4009, "Interface.lvclass"=w4008, "Channel in"=w3993) -> ("error out"=w4015:errorcluster, "Channel out"=w4016:refnum<class "Channel.lvclass">)  [unwired: 7 in]
                n1780 = call "Write section_name.vi"("error in (no error)"=w4015, "section_name"="CCD_ACS3", "Channel in"=w4016) -> ("error out"=w4013:errorcluster, "Channel out"=w4019:refnum<class "Channel.lvclass">)  [unwired: 7 in]
                n1781 = call-dynamic "save config.vi"("error in (no error)"=w4013, "file config"="lastsaved.cfg", "Channel in"=w4019) -> ("error out"=w4014:errorcluster, "Channel out"=w4020:refnum<class "Channel.lvclass">)  [unwired: 7 in]
                n1782 = call-dynamic "Read State Machine.vi"("error in (no error)"=w4014, "Device in"=w4020) -> ("error out"=w4010:errorcluster, "State Machine.lvclass"=w4022:refnum<class "State Machine.lvclass">, "Device out"=w4021:refnum<class "Channel.lvclass">)  [unwired: 7 in]
                n1783 = call-dynamic "Write State.vi"("error in (no error)"=w4010, "State"=60, "State Machine in"=w4022) -> ("error out"=w4011:errorcluster, "State Machine out"=w4023:refnum<class "State Machine.lvclass">)  [unwired: 7 in]
                n1784 = call-dynamic "Write State Machine.vi"("error in (no error)"=w4011, "State Machine.lvclass"=w4023, "Device in"=w4021) -> ("error out"=w4025:errorcluster, "Device out"=w4024:refnum<class "Channel.lvclass">)  [unwired: 7 in]
                n1785 = call-dynamic "Write Channel.vi"("error in (no error)"=w4025, "Channel.lvclass"=w4024, "Acquisition in"=w3994) -> ("error out"=w3989:errorcluster, "Acquisition out"=w3990:refnum<class "Acquisition.lvclass">)  [unwired: 7 in]
              }
            }
            n1786 = case shown="True" w3921 {
              tunnel: w3923 -> [w3949 w3953]
              tunnel: w3922 -> [w3948 w3952]
              tunnel: [w3949 w3951] -> w3936
              tunnel: [w3948 w3950] -> w3935
              frame False {
              }
              frame True {
                # "nome do arquivo .cfg"
                # "seção no arquivo .cfg"
                # "closed"
                n1787 = call-dynamic "Read Channel.vi"("error in (no error)"=w3952, "Acquisition in"=w3953) -> ("error out"=w3983:errorcluster, "Channel.lvclass"=w3984:refnum<class "Channel.lvclass">, "Acquisition out"=w3985:refnum<class "Acquisition.lvclass">)  [unwired: 7 in]
                n1788 = call-dynamic "Read Interface.vi"("error in (no error)"=w3983, "Channel in"=w3984) -> ("error out"=w3975:errorcluster, "Interface.lvclass"=w3974:refnum<class "Interface.lvclass">, "Channel out"=w3986:refnum<class "Channel.lvclass">)  [unwired: 7 in]
                n1789 = call-dynamic "Get CCD_Config.vi"("error in (no error)"=w3975, "Interface in"=w3974) -> ("error out"=w3978:errorcluster, "output cluster"=w3979:T24, "Interface out"=w3973:refnum<class "Interface.lvclass">)  [unwired: 7 in]
                n1790 = Bundle By Name(cluster=w3979, "SHUTTER_MODE"=u8 2) -> (w3977:T24)
                n1791 = call-dynamic "Set CCD_Config.vi"("error in (no error)"=w3978, "input cluster"=w3977, "Interface in"=w3973) -> ("error out"=w3980:errorcluster, "Interface out"=w3972:refnum<class "Interface.lvclass">)  [unwired: 7 in]
                n1792 = Flatten To String(anything=w3977, error in (no error)=w3980) -> (data string=w3982:string, error out=w3981:errorcluster)  [unwired: 2 in, 1 out]
                n1793 = call "Write flatted cluster.vi"("error in (no error)"=w3981, "flatted cluster"=w3982, "Interface in"=w3972) -> ("error out"=w3970:errorcluster, "Interface out"=w3971:refnum<class "Interface.lvclass">)  [unwired: 7 in]
                n1794 = call-dynamic "Write Interface.vi"("error in (no error)"=w3970, "Interface.lvclass"=w3971, "Channel in"=w3986) -> ("error out"=w3964:errorcluster, "Channel out"=w3963:refnum<class "Channel.lvclass">)  [unwired: 7 in]
                n1795 = call "Write section_name.vi"("error in (no error)"=w3964, "section_name"="CCD_ACS4", "Channel in"=w3963) -> ("error out"=w3966:errorcluster, "Channel out"=w3960:refnum<class "Channel.lvclass">)  [unwired: 7 in]
                n1796 = call-dynamic "save config.vi"("error in (no error)"=w3966, "file config"="lastsaved.cfg", "Channel in"=w3960) -> ("error out"=w3965:errorcluster, "Channel out"=w3959:refnum<class "Channel.lvclass">)  [unwired: 7 in]
                n1797 = call-dynamic "Read State Machine.vi"("error in (no error)"=w3965, "Device in"=w3959) -> ("error out"=w3969:errorcluster, "State Machine.lvclass"=w3957:refnum<class "State Machine.lvclass">, "Device out"=w3958:refnum<class "Channel.lvclass">)  [unwired: 7 in]
                n1798 = call-dynamic "Write State.vi"("error in (no error)"=w3969, "State"=60, "State Machine in"=w3957) -> ("error out"=w3968:errorcluster, "State Machine out"=w3956:refnum<class "State Machine.lvclass">)  [unwired: 7 in]
                n1799 = call-dynamic "Write State Machine.vi"("error in (no error)"=w3968, "State Machine.lvclass"=w3956, "Device in"=w3958) -> ("error out"=w3954:errorcluster, "Device out"=w3955:refnum<class "Channel.lvclass">)  [unwired: 7 in]
                n1800 = call-dynamic "Write Channel.vi"("error in (no error)"=w3954, "Channel.lvclass"=w3955, "Acquisition in"=w3985) -> ("error out"=w3950:errorcluster, "Acquisition out"=w3951:refnum<class "Acquisition.lvclass">)  [unwired: 7 in]
              }
            }
            n1801 = disable-structure shown="Enabled" {
              frame Disabled {
                # "closed"
                n1802 = local read "Input Cluster"() -> (w3945:T5)
                n1803 = Unbundle By Name(w3945) -> ("Parameters"=w3946:T23)
                n1804 = Bundle By Name(cluster=w3946, "Shutter\nMode"=u16 2 ("Shutter\nMode")) -> (w3943:T23)
                n1805 = Bundle By Name(cluster=w3945, "Parameters"=w3943) -> (w3944:T5)
                n1806 = local write "Input Cluster"(w3944) -> ()
              }
              frame Enabled {
              }
            }
          }
          frame "OBJECT", Default {
            # "OBJECT, DFLAT,SFLAT and FOCUS: Shutter automatically open."
            n1807 = call "Read connection.vi"("error in (no error)"=w4109, "Server in"=w4110) -> ("error out"=w4116:errorcluster, "connection"=w4115:bool, "Server out"=w4117:refnum<class "Acquisition.lvclass">)  [unwired: 7 in]
            n1808 = call "Read connection.vi"("error in (no error)"=w4111, "Server in"=w4112) -> ("error out"=w4119:errorcluster, "connection"=w4118:bool, "Server out"=w4120:refnum<class "Acquisition.lvclass">)  [unwired: 7 in]
            n1809 = call "Read connection.vi"("error in (no error)"=w4113, "Server in"=w4114) -> ("error out"=w4122:errorcluster, "connection"=w4121:bool, "Server out"=w4123:refnum<class "Acquisition.lvclass">)  [unwired: 7 in]
            n1810 = call "Read connection.vi"("error in (no error)"=w4127, "Server in"=w4128) -> ("error out"=w4125:errorcluster, "connection"=w4124:bool, "Server out"=w4126:refnum<class "Acquisition.lvclass">)  [unwired: 7 in]
            n1811 = case shown="True" w4121 {
              tunnel: w4123 -> [w4267 w4296]
              tunnel: w4122 -> [w4266 w4295]
              tunnel: [w4267 w4294] -> w4134
              tunnel: [w4266 w4293] -> w4133
              tunnel: w4108 -> [_ w4272]
              tunnel: w4107 -> [_ w4271]
              tunnel: w4106 -> [_ w4270]
              tunnel: w4105 -> [_ w4269]
              tunnel: w4104 -> [_ w4268]
              frame False {
              }
              frame True {
                # "nome do arquivo .cfg"
                # "seção no arquivo .cfg"
                # "open"
                n1812 = call-dynamic "Read Channel.vi"("error in (no error)"=w4295, "Acquisition in"=w4296) -> ("error out"=w4300:errorcluster, "Channel.lvclass"=w4299:refnum<class "Channel.lvclass">, "Acquisition out"=w4298:refnum<class "Acquisition.lvclass">)  [unwired: 7 in]
                n1813 = call-dynamic "Read Interface.vi"("error in (no error)"=w4300, "Channel in"=w4299) -> ("error out"=w4308:errorcluster, "Interface.lvclass"=w4309:refnum<class "Interface.lvclass">, "Channel out"=w4297:refnum<class "Channel.lvclass">)  [unwired: 7 in]
                n1814 = call-dynamic "Get CCD_Config.vi"("error in (no error)"=w4308, "Interface in"=w4309) -> ("error out"=w4305:errorcluster, "output cluster"=w4304:T24, "Interface out"=w4310:refnum<class "Interface.lvclass">)  [unwired: 7 in]
                n1815 = Bundle By Name(cluster=w4304, "SHUTTER_MODE"=u8 1) -> (w4306:T24)
                n1816 = call-dynamic "Set CCD_Config.vi"("error in (no error)"=w4305, "input cluster"=w4306, "Interface in"=w4310) -> ("error out"=w4303:errorcluster, "Interface out"=w4311:refnum<class "Interface.lvclass">)  [unwired: 7 in]
                n1817 = Flatten To String(anything=w4306, error in (no error)=w4303) -> (data string=w4301:string, error out=w4302:errorcluster)  [unwired: 2 in, 1 out]
                n1818 = call "Write flatted cluster.vi"("error in (no error)"=w4302, "flatted cluster"=w4301, "Interface in"=w4311) -> ("error out"=w4313:errorcluster, "Interface out"=w4312:refnum<class "Interface.lvclass">)  [unwired: 7 in]
                n1819 = call-dynamic "Write Interface.vi"("error in (no error)"=w4313, "Interface.lvclass"=w4312, "Channel in"=w4297) -> ("error out"=w4318:errorcluster, "Channel out"=w4319:refnum<class "Channel.lvclass">)  [unwired: 7 in]
                n1820 = call "Write section_name.vi"("error in (no error)"=w4318, "section_name"="CCD_ACS2", "Channel in"=w4319) -> ("error out"=w4317:errorcluster, "Channel out"=w4322:refnum<class "Channel.lvclass">)  [unwired: 7 in]
